vi "simple_adc.vi"() -> ()   [LabVIEW 2017]
uses:
  lib/libbuddy/bindings/labview/utility_vi/buddy.lvlib
panel:
  out "handle":u64
  out "function return 2":i32
  out "BOOL_CH8":bool=TRUE
  out "BOOL_CH7":bool=TRUE
  out "BOOL_CH6":bool=TRUE
  out "BOOL_CH5":bool=TRUE
  out "BOOL_CH4":bool=TRUE
  out "BOOL_CH3":bool=TRUE
  out "BOOL_CH2":bool=TRUE
  out "BOOL_CH1":bool=TRUE
  out "function return":i32
  out "packet out":T1
  out "Waveform Chart Using Bundle":T1(graph)
  out "Iterations":i32
  out "Time":dbl
  out "ADC Sample Time":dbl
  in  "stop":bool
  out "timing":cluster{"period":u32, "averaging":u8}
  in  "ADC Sample Rate (Hz)":dbl=1000.0
  out "fw_info out":T2
  in  "timing":cluster{"period":u32, "averaging":u8}={"period"=1000000, "averaging"=1}
  in  "runtime":T3={"dac_power"=0, "dac_ref"=0, "adc_ref"=2, "adc_gain"=0}
  in  "general":T4={"function"=3, "mode"=0, "channel_mask"=255, "resolution"=1}
  out "str_serial":string
  out "str_mfr":string
  out "str_product":string
  out "str_index_1":string
  # "CONFIGURATION"
  # "DEVICE INFO"
  # "ADC VALUES"
  # "CH1"
  # "CH2"
  # "CH3"
  # "CH4"
  # "CH5"
  # "CH6"
  # "CH7"
  # "CH8"
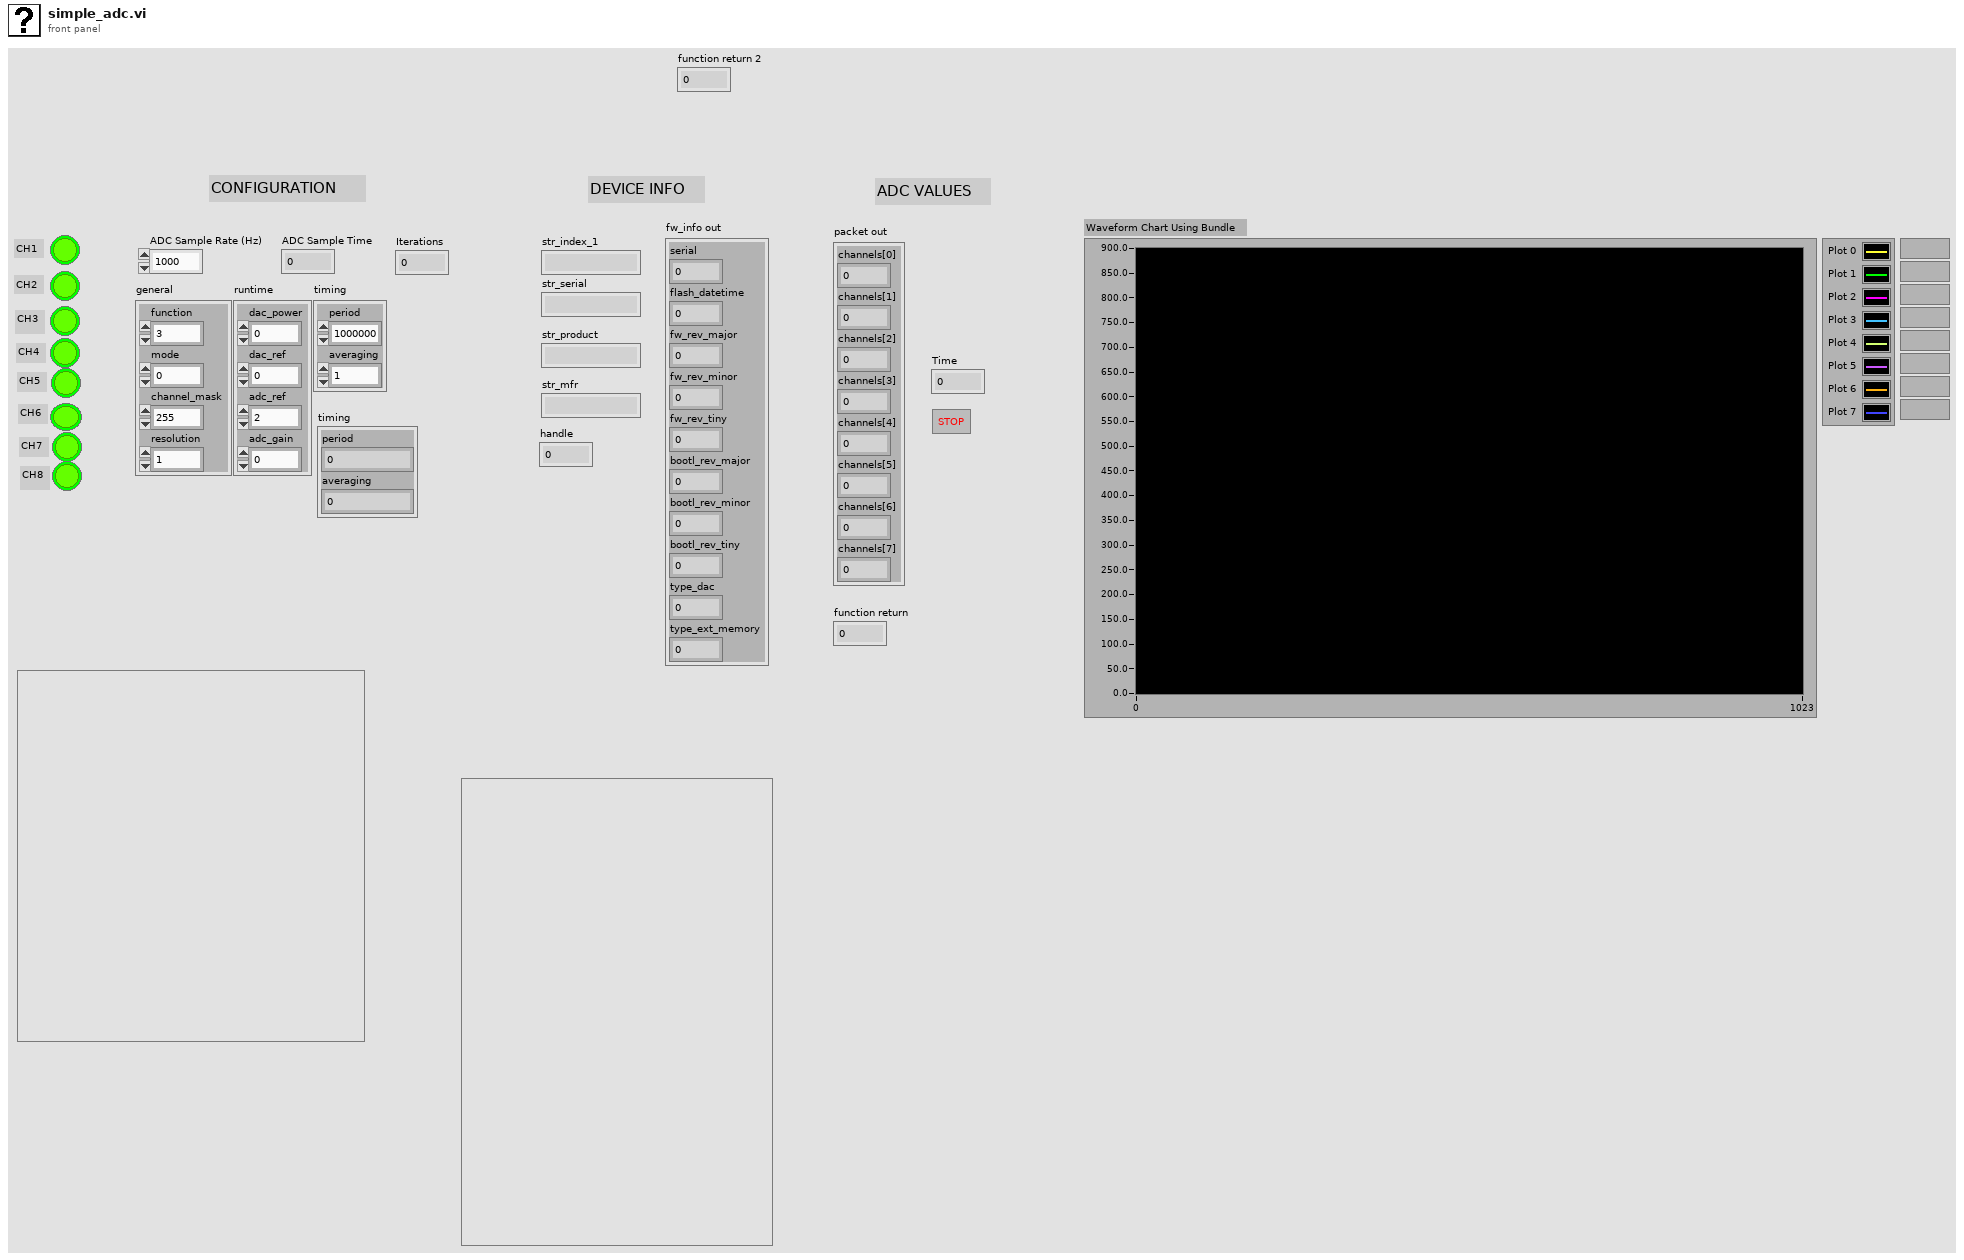
[diagram p1: front panel]
types:
  T1 = cluster{"channels[0]":u16, "channels[1]":u16, "channels[2]":u16, "channels[3]":u16, "channels[4]":u16, "channels[5]":u16, "channels[6]":u16, "channels[7]":u16}
  T2 = cluster{"serial":u32, "flash_datetime":u32, "fw_rev_major":u8, "fw_rev_minor":u8, "fw_rev_tiny":u8, "bootl_rev_major":u8, "bootl_rev_minor":u8, "bootl_rev_tiny":u8, "type_dac":u8, "type_ext_memory":u8}
  T3 = cluster{"dac_power":u8, "dac_ref":u8, "adc_ref":u8, "adc_gain":u8}
  T4 = cluster{"function":u8, "mode":u8, "channel_mask":u8, "resolution":u8}
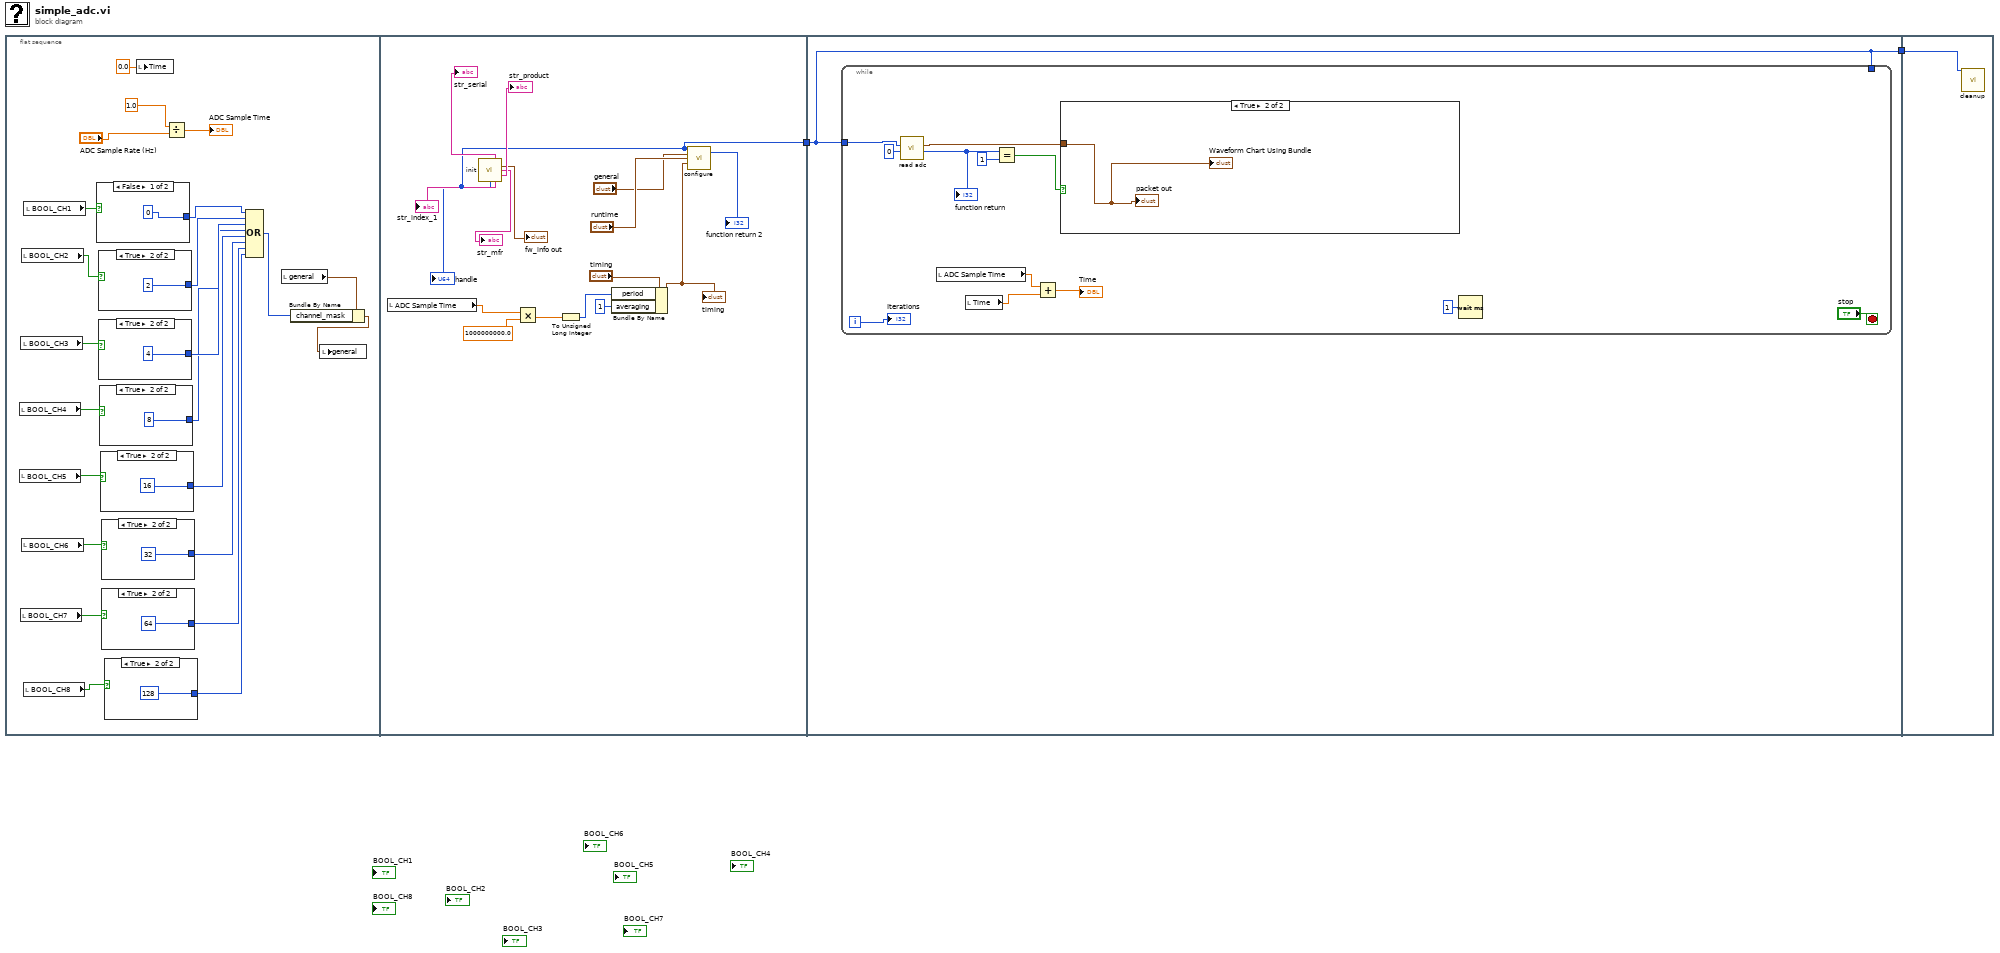
[diagram p0: block diagram]
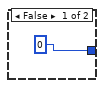
[diagram p2: hidden frame]
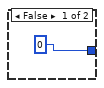
[diagram p3: hidden frame]
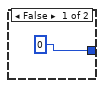
[diagram p4: hidden frame]
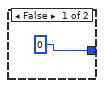
[diagram p5: hidden frame]
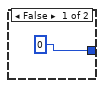
[diagram p6: hidden frame]
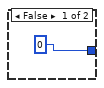
[diagram p7: hidden frame]
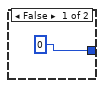
[diagram p8: hidden frame]
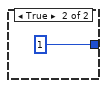
[diagram p9: hidden frame]
diagram:
  n1 = flat-sequence {
    tunnel: [w42] -> w1
    tunnel: [w58] -> w2
    tunnel: w1 -> [w58]
    tunnel: w2 -> [w72]
    frame #0 {
      n2 = local read "BOOL_CH4"() -> (w16:bool)
      n3 = local read "BOOL_CH5"() -> (w15:bool)
      n4 = local read "BOOL_CH7"() -> (w13:bool)
      n5 = local read "BOOL_CH3"() -> (w17:bool)
      n6 = local read "BOOL_CH2"() -> (w18:bool)
      n7 = local read "BOOL_CH6"() -> (w14:bool)
      n8 = local read "BOOL_CH8"() -> (w12:bool)
      n9 = local read "BOOL_CH1"() -> (w21:bool)
      n10 = case shown="False" w21 {
        tunnel: [u8 0 ("averaging") u8 1 ("averaging")] -> w20
        frame False {
        }
        frame True {
        }
      }
      n11 = case shown="True" w18 {
        tunnel: [u8 0 ("averaging") u8 2 ("averaging")] -> w19
        frame False {
        }
        frame True {
        }
      }
      n12 = case shown="True" w17 {
        tunnel: [u8 0 ("averaging") u8 4 ("averaging")] -> w11
        frame False {
        }
        frame True {
        }
      }
      n13 = case shown="True" w16 {
        tunnel: [u8 0 ("averaging") u8 8 ("averaging")] -> w10
        frame False {
        }
        frame True {
        }
      }
      n14 = case shown="True" w15 {
        tunnel: [u8 0 ("averaging") u8 16 ("averaging")] -> w9
        frame False {
        }
        frame True {
        }
      }
      n15 = case shown="True" w14 {
        tunnel: [u8 0 ("averaging") u8 32 ("averaging")] -> w8
        frame False {
        }
        frame True {
        }
      }
      n16 = case shown="True" w13 {
        tunnel: [u8 0 ("averaging") u8 64 ("averaging")] -> w7
        frame False {
        }
        frame True {
        }
      }
      n17 = case shown="True" w12 {
        tunnel: [u8 0 ("averaging") u8 128 ("averaging")] -> w6
        frame False {
        }
        frame True {
        }
      }
      n18 = local write "Time"(0.0 ("Time")) -> ()
      n19 = Divide(x=1.0, y="ADC Sample Rate (Hz)") -> (x/y=→"ADC Sample Time":dbl)
      n20 = Compound Arithmetic op=OR(w20, w19, w11, w10, w9, w8, w7, w6) -> (w4:u8)
      n21 = local read "general"() -> (w5:T4)
      n22 = Bundle By Name(cluster=w5, "channel_mask"=w4) -> (w3:T4)
      n23 = local write "general"(w3) -> ()
    }
    frame #1 {
      n24 = local read "ADC Sample Time"() -> (w44:dbl)
      n25 = call "init.vi"() -> ("str_serial"=→"str_serial":string, "fw_info out"=→"fw_info out":T2, "str_mfr"=→"str_mfr":string, "str_product"=→"str_product":string, "return type"=w42:u64, "str_index_1"=→"str_index_1":string)  [unwired: 8 in, 2 out]
      "handle" <- w42
      n26 = Multiply(x=w44, y=1000000000.0) -> (x*y=w47:dbl)
      n27 = To Unsigned Long Integer(number=w47) -> (unsigned 32bit integer=w46:u32)
      n28 = Bundle By Name(cluster="timing", "period"=w46, "averaging"=u8 1) -> (w49:cluster{"period":u32, "averaging":u8})
      "timing" <- w49
      n29 = call "configure.vi"("handle in"=w42, "general"="general", "runtime"="runtime", "timing"=w49) -> ("function return"=→"function return 2":i32)  [unwired: 7 in, 4 out]
    }
    frame #2 {
      n30 = while {
        tunnel: w58 -> [_]
        tunnel: w58 -> [w59]
        i -> [w66]
        stop <- "stop" stop-if-true
        n31 = call "read adc.vi"("streaming"=0, "handle"=w59) -> ("function return"=w64:i32, "packet out"=w61:T1)  [unwired: 7 in, 1 out]
        "function return" <- w64
        n32 = local read "ADC Sample Time"() -> (w67:dbl)
        n33 = local read "Time"() -> (w68:dbl)
        n34 = Equal?(x=w64, y=1) -> (x = y?=w62:bool)
        n35 = Add(x=w67, y=w68) -> (x+y=→"Time":dbl)
        n36 = case shown="True" w62 {
          tunnel: w61 -> [_ w71]
          frame False {
          }
          frame True {
            "packet out" <- w71
            "Waveform Chart Using Bundle" <- w71
          }
        }
        n37 = Wait (ms)(milliseconds to wait=u32 1) -> ()  [unwired: 1 out]
        "Iterations" <- w66
      }
    }
    frame #3 {
      n38 = call "cleanup.vi"("handle"=w72) -> ()  [unwired: 13 in, 2 out]
    }
  }
